vi "Destroy.vi"(8 "error in (no error)":errorcluster, 11 "Client in":refnum<class "Client.lvclass">) -> (0 "error out":errorcluster, 3 "Client out":refnum<class "Client.lvclass">)   [LabVIEW 2013, in "MQTT Server.lvlib" / "Client.lvclass"]
uses:
  Client.lvclass
  MQTT_Base/MQTT_Base.lvclass
  Client.lvclass/Client.ctl
  Server/Session/Session.lvclass
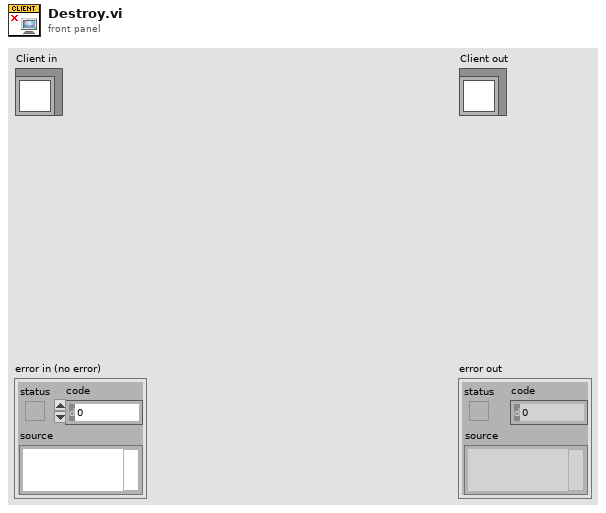
[diagram p1: front panel]
types:
  T1 = typedef "MQTT Server.lvlib/Client.lvclass/Public Events -- cluster.ctl" = cluster{"Connection Status":refnum<user-event>, "Connected":refnum<user-event>, "Application Message":refnum<user-event>}
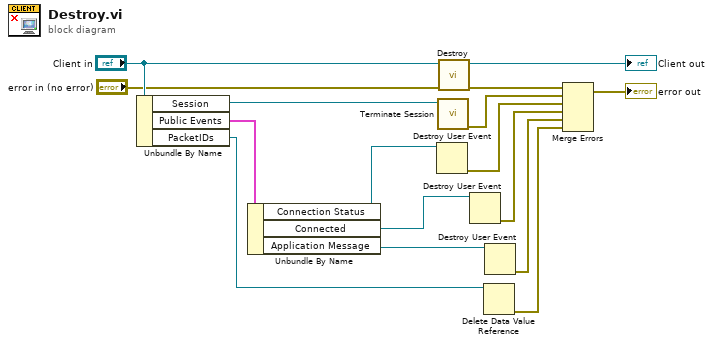
[diagram p0: block diagram]
diagram:
  n1 = Unbundle By Name("Client in") -> ("Session"=w12:refnum<class "Session.lvclass">, "Public Events"=w8:T1, "PacketIDs"=w4:refnum<data-value>)
  n2 = Unbundle By Name(w8) -> ("Connection Status"=w7:refnum<user-event>, "Connected"=w6:refnum<user-event>, "Application Message"=w5:refnum<user-event>)
  n3 = Destroy User Event(user event=w7) -> (error out=w9:errorcluster)  [unwired: 1 in]
  n4 = call "Terminate Session.vi"("Session in"=w12) -> ("error out"=w11:errorcluster)  [unwired: 8 in, 2 out]
  n5 = call-parent "Destroy.vi"("error in (no error)"="error in (no error)", "MQTT_Base in"="Client in") -> ("error out"=w15:errorcluster, "MQTT_Base out"=→"Client out":refnum<class "Client.lvclass">)  [unwired: 8 in]
  n6 = Destroy User Event(user event=w6) -> (error out=w2:errorcluster)  [unwired: 1 in]
  n7 = Delete Data Value Reference(data value reference=w4) -> (error out=w3:errorcluster)  [unwired: 1 in, 1 out]
  n8 = Destroy User Event(user event=w5) -> (error out=w1:errorcluster)  [unwired: 1 in]
  n9 = Merge Errors(w15, w11, w9, w2, w1, w3) -> (→"error out":errorcluster)
